vi "GlobalTimerAcquisition.vi"() -> ()   [LabVIEW 2022 SP3]
panel:
  out "Numeric":dbl
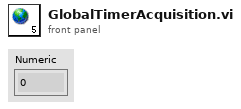
[diagram p1: front panel]
diagram:
